vi "9.4.vi"() -> ()   [LabVIEW 2019]
panel:
  in  "Enum":enum16{"(x*y)", "(x-y)", "(x/y)", "(x+y)"}(ring)
  out "Numeric":dbl
  in  "y":dbl
  in  "x":dbl
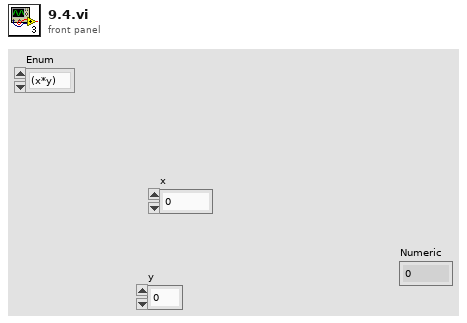
[diagram p1: front panel]
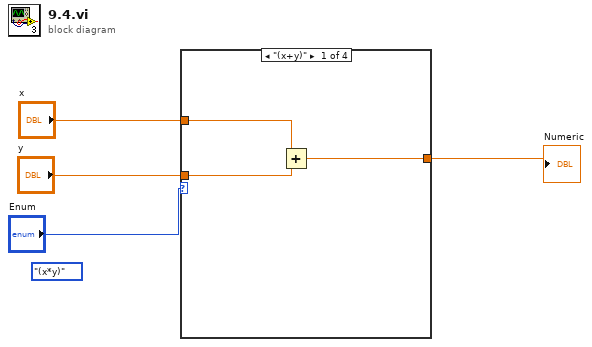
[diagram p0: block diagram]
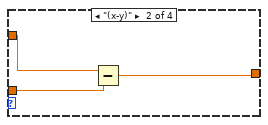
[diagram p2: hidden frame]
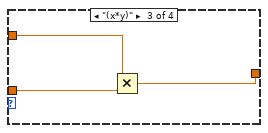
[diagram p3: hidden frame]
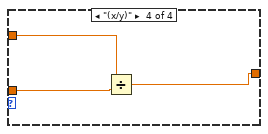
[diagram p4: hidden frame]
diagram:
  (unwired) enum16{"(x*y)", "(x-y)", "(x/y)", "(x+y)"}."(x*y)"
  n1 = case shown="\"(x+y)\"" "Enum" {
    tunnel: "x" -> [w7 w9 w12 w15]
    tunnel: "y" -> [w6 w8 w11 w14]
    tunnel: [w5 w10 w13 w16] -> w2
    frame "(x+y)" {
      n2 = Add(x=w7, y=w6) -> (x+y=w5:dbl)
    }
    frame "(x-y)" {
      n3 = Subtract(x=w9, y=w8) -> (x-y=w10:dbl)
    }
    frame "(x*y)" {
      n4 = Multiply(x=w12, y=w11) -> (x*y=w13:dbl)
    }
    frame "(x/y)" {
      n5 = Divide(x=w15, y=w14) -> (x/y=w16:dbl)
    }
  }
  "Numeric" <- w2
